vi "LockinDAQ.getREF.vi"(8 "error in (no error)":errorcluster, 10 "getREF":T1, 11 "LockinDAQ":refnum<class "LockinDAQ.lvclass">) -> (0 "error out":errorcluster, 3 "LockinDAQ out":refnum<class "LockinDAQ.lvclass">)   [LabVIEW 2016, in "LockinDAQ.lvclass"]
doc: "---------------------------------------------------------------\nJKI State Machine Objects™\nhttp://jki.net/state-machine-objects/\nCopyright (C) 2005-2015, JKI <info@jki.net>\nALL RIGHTS RESERVEDJKI State Machine Objects (SMO) 1.0.0.4\nJKI - JKI\nCopyright (c) 2015, JKI"
uses:
  LockinDAQ.lvclass
  Typedefs/PublicEvents--LockinDAQ.getREF.ctl
  LockinDAQ.lvclass/LockinDAQ.ctl
panel:
  # "For instructions on how to use the JKI State Machine Objects, examples and video tutorials, visit:\nhttp://jki.net/state-machine-objects/\n\nJKI State Machine Objects™\nhttp://jki.net/state-machine-objects/\nCopyright (C) 2005-2015, JKI <info@jki.net>\nALL RIGHTS RESERVED"
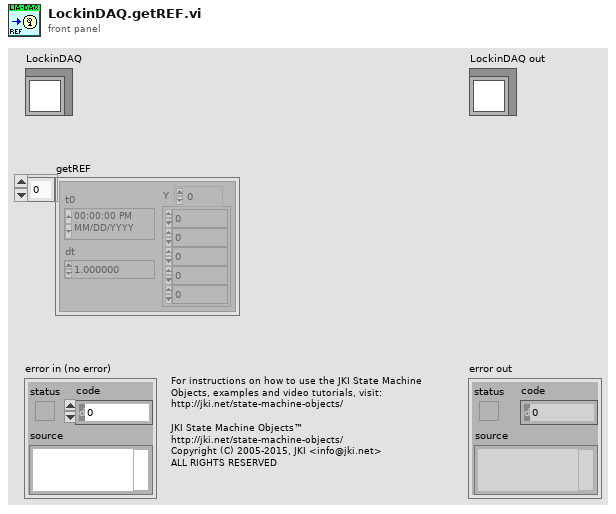
[diagram p1: front panel]
types:
  T1 = typedef "LockinDAQ.lvclass/PublicEvents--LockinDAQ.getREF.ctl" = waveform(dbl)[]
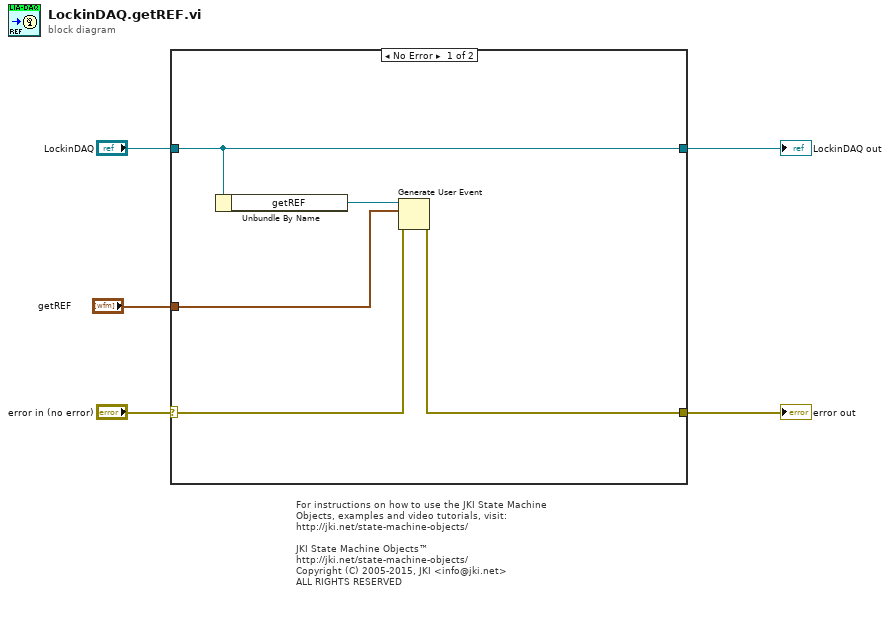
[diagram p0: block diagram]
diagram:
  # "For instructions on how to use the JKI State Machine Objects, examples and video tutorials, visit:\nhttp://jki.net/state-machine-objects/\n\nJKI State Machine Objects™\nhttp://jki.net/state-machine-objects/\nCopyright (C) 2005-2015, JKI <info@jki.net>\nALL RIGHTS RESERVED"
  n1 = case shown="No Error" "error in (no error)" {
    selector: "error in (no error)" -> [w10 w12]
    tunnel: [w7 w12] -> w4
    tunnel: [w6 w11] -> w5
    tunnel: "LockinDAQ" -> [w6 w11]
    tunnel: "getREF" -> [w9 _]
    frame No Error {
      n2 = Unbundle By Name(w6) -> ("getREF"=w8:refnum<user-event>)
      n3 = Generate User Event(user event=w8, event data cluster=w9, error in=w10) -> (error out=w7:errorcluster)  [unwired: 1 in, 1 out]
    }
    frame Error {
    }
  }
  "error out" <- w4
  "LockinDAQ out" <- w5
